vi "FTW-System-CurrentMemoryStatistics.vi"(11 "error in":errorcluster) -> (4 "DS Bytes Allocated":i64 format="%_4pbytes", 15 "error out":errorcluster)   [LabVIEW 2015]
panel:
  # "Inputs"
  # "Outputs"
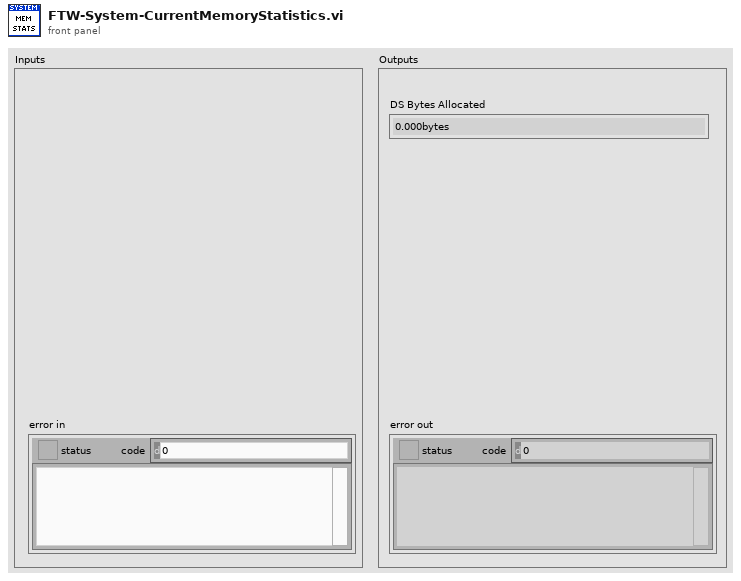
[diagram p1: front panel]
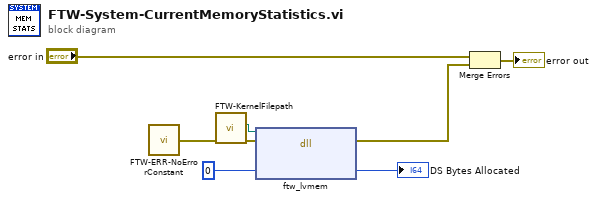
[diagram p0: block diagram]
diagram:
  n1 = call "FTW-ERR-NoErrorConstant.vi"() -> ("no error"=w2:errorcluster)
  n2 = call "FTW-KernelFilepath.vi"("error in"=w2) -> ("error out"=w3:errorcluster, "Library Filepath"=w1:path)  [unwired: 8 in, 1 out]
  n3 = dll-call lib="?" fn="ftw_lvmem"(path in=w1, error in=w3, "Bytes Allocated"=i64 0 ("DS Max Available Handle Size")) -> (error out=w4:errorcluster, "Bytes Allocated"=→"DS Bytes Allocated":i64)  [unwired: 2 in, 1 out]
  n4 = Merge Errors("error in", w4) -> (→"error out":errorcluster)
